vi "Test Suite from Test Case Path Status Correct.vi"(8 "error in (no error)":errorcluster, 11 "Test Case In":refnum<class "LUnit Test Suite Tests.lvclass">) -> (0 "error out":errorcluster, 3 "Test Case Out":refnum<class "LUnit Test Suite Tests.lvclass">)   [LabVIEW 2020, in "LUnit Test Suite Tests.lvclass"]
uses:
  LUnit Test Suite Tests.lvclass
  C:/Program Files (x86)/National Instruments/LabVIEW 2020/vi.lib/Astemes/LUnit/Test Case.lvclass
  Test Doubles/Test Case Test Double/Test Case Test Double.lvclass
  source/Core/Result/Status.ctl
  <vilib>/Astemes/LUnit/Test Case.lvclass/Test Case.ctl
  b74e4934-f044-4222-b3dd-fc90e6c1bd4f.vi
  <vilib>/Astemes/LUnit/Append Pass Result.vi
  <vilib>/Astemes/LUnit/Append Fail Result.vi
  <vilib>/Astemes/LUnit/Compare Variants.vi
  <vilib>/Astemes/LUnit/Describe Comparison.vi
  <vilib>/Astemes/LUnit/Variant to string.vi
  source/API/LUnit Test Suite/LUnit Test Suite.lvclass
  C:/git/astemes-lunit/source/Core/Runnable/Runnable.lvclass
  <vilib>/Utility/Data Type/Get Type Information.vi
  <vilib>/Utility/LVClass/Get LV Class Name.vi
  source/Core/Result/Result.lvlib
  source/Core/Runnable/Runnable.lvclass
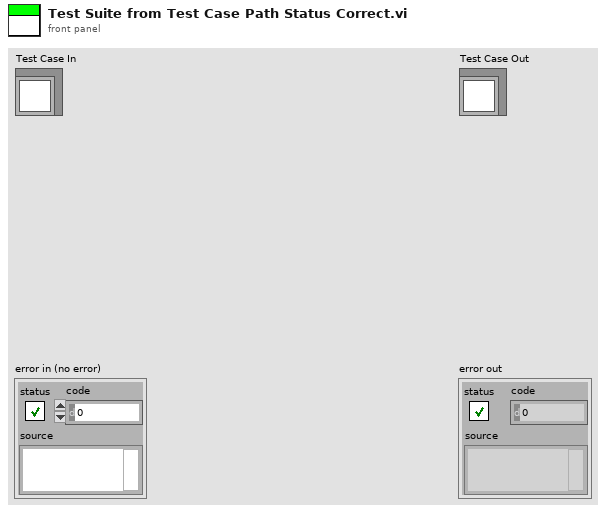
[diagram p1: front panel]
types:
  T1 = typedef "Result.lvlib/Status.ctl" = enum16{"", "Passed", "Failed", "Error", "Skipped", "Setup Error", "Broken", "Teardown Error"}
  T2 = typedef "Result.lvlib/Result.ctl" = cluster{"Name":string, "Message":string, "Description":string, "Status":T1, "Result Type":T3, "Execution Time":dbl}
  T3 = typedef "Result.lvlib/Type.ctl" = enum16{"Test Case", "Test Suite", "Test Run", "Pass", "Fail", "Skip", "Pass if", "Fail if", "Pass if Error", "Fail if Error", "Pass if Equal", "Fail if Equal"}
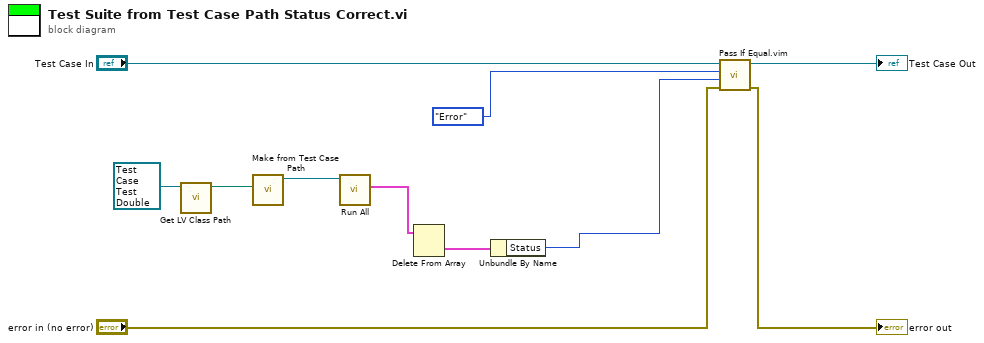
[diagram p0: block diagram]
diagram:
  n1 = call <vilib>:"Get LV Class Path.vi"("object"=refnum<class "Test Case Test Double.lvclass"> refnum ("LUnit Test Case V2 Test Double.lvclass")) -> ("class path"=w1:path)  [unwired: 9 in, 1 out]
  n2 = call "Make from Test Case Path.vi"("Test Case"=w1) -> ("LUnit Test Suite Out"=w6:refnum<class "LUnit Test Suite.lvclass">)  [unwired: 9 in, 1 out]
  n3 = call "Run All.vi"("Runnable In"=w6) -> ("Results"=w5:T2[])  [unwired: 9 in, 1 out]
  n4 = Delete From Array(array=w5) -> (deleted portion=w4:T2)  [unwired: 2 in, 1 out]
  n5 = Unbundle By Name(w4) -> ("Status"=w3:T1)
  n6 = call "Pass If Equal.vim"("error in (no error)"="error in (no error)", "Actual"=w3, "Expected"=Status."Error" ("Status"), "LUnit Test Case In"="Test Case In") -> ("error out"=→"error out":errorcluster, "LUnit Test Case Out"=→"Test Case Out":refnum<class "LUnit Test Suite Tests.lvclass">)  [unwired: 6 in]
